vi "Input 3.vi"(8 "error in (no error)":errorcluster, 11 "Node Ptr":T2 format="%.0x") -> (0 "error out":errorcluster)   [LabVIEW 2019, in "Software Multi-Plex System Explorer.lvlib"]
uses:
  Software Multi-Plex System Explorer.lvlib
  <vilib>/NI VeriStand/Custom Device API/Custom Device Item Ref.ctl
  <vilib>/NI VeriStand/UI Controls/Tree and Alias Browser/Tree Alias Browser Display.ctl
  NationalInstruments.VeriStand.SystemStorageUI
  NationalInstruments.VeriStand.SystemStorage
  <vilib>/NI VeriStand/Custom Device API/Custom Device API.lvlib
  <vilib>/NI VeriStand/UI Controls/Tree and Alias Browser/NI_VS UI Tree Alias Browser.lvlib
panel:
  in  "Map Input":bool
  out "Input Path":string
  in  "Tree Browser":T1
  in  "Specific Header":cluster{"Section Name":string}={"Section Name"="Specify Input 3 Channel Source"}
  in  "General Header":cluster{"Section Name":string}={"Section Name"="Software Multi-Plex Channel Input 3 Settings"}
  in  "Description":string
  in  "Name":string
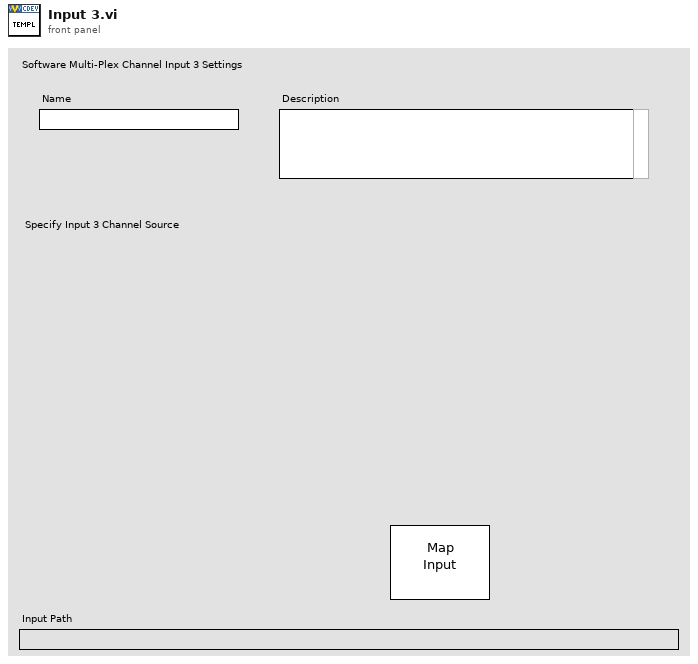
[diagram p1: front panel]
types:
  T1 = typedef "NI_VS UI Tree Alias Browser.lvlib/Tree Alias Browser Display.ctl" = refnum<k24>
  T2 = typedef "Custom Device API.lvlib/Custom Device Item Ref.ctl" = u64
  T3 = typedef "NI_VS UI Tree Alias Browser.lvlib/Callback Type.ctl" = cluster{"Net Callbacks":refnum<k27>[], "Event":T4}
  T4 = typedef "NI_VS UI Tree Alias Browser.lvlib/Net Event Data Ref.ctl" = refnum<user-event>
  T5 = typedef "NI_VS UI Tree Alias Browser.lvlib/Tree Alias Browser Ref.ctl" = refnum<k24>
  T6 = typedef "Custom Device API.lvlib/Custom Device Item Info.ctl" = cluster{"Name":string, "Is Channel":bool, "GUID":string, "Is Waveform":bool}
  T7 = typedef "Custom Device API.lvlib/Custom Device Commands.ctl" = enum16{"Default", "Item renamed", "Shutdown", "Dynamic button pressed"}
  T8 = typedef "NI_VS UI Tree Alias Browser.lvlib/Net Event.ctl" = enum16{"SelectedItem", "DblClick"}
  T9 = typedef "Custom Device API.lvlib/Custom Device Pointer.ctl" = refnum<k24>
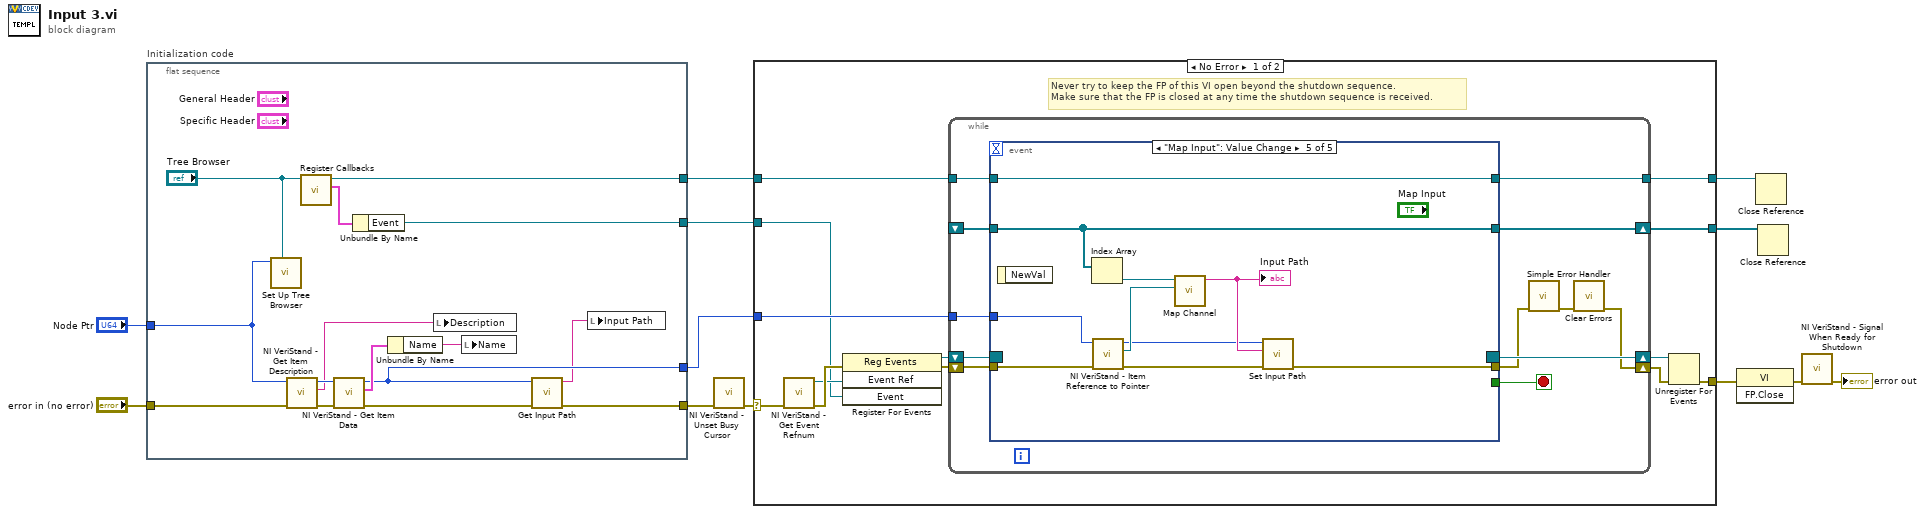
[diagram p0: block diagram]
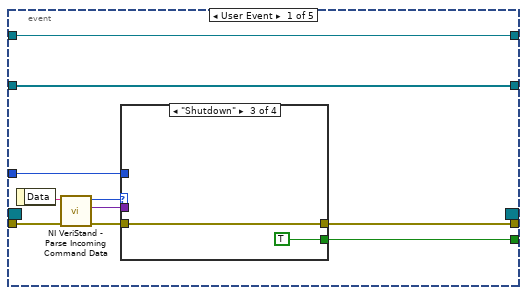
[diagram p2: hidden frame]
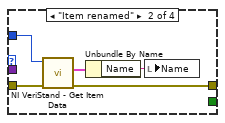
[diagram p4: hidden frame]
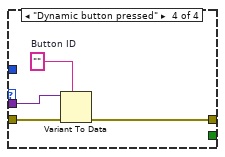
[diagram p5: hidden frame]
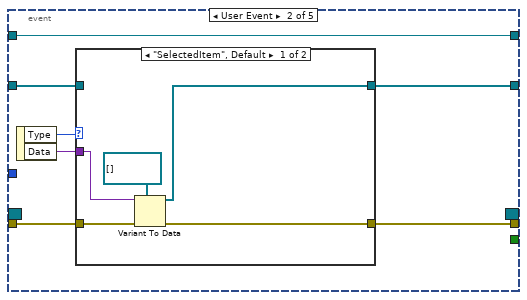
[diagram p6: hidden frame]
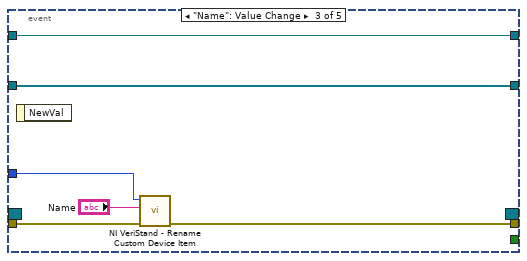
[diagram p8: hidden frame]
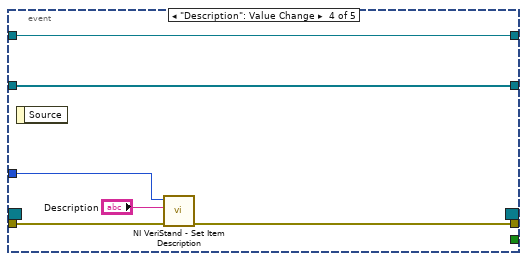
[diagram p9: hidden frame]
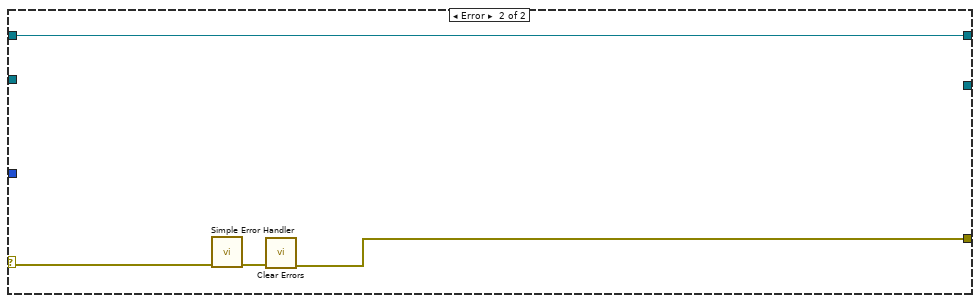
[diagram p10: hidden frame]
diagram:
  n1 = flat-sequence "Initialization code" {
    tunnel: "error in (no error)" -> [w22]
    tunnel: "Node Ptr" -> [w21]
    tunnel: [w16] -> w8
    tunnel: [w14] -> w5
    tunnel: [w19] -> w4
    tunnel: [w17] -> w2
    frame #0 {
      n2 = call "Set Up Tree Browser.vi"("Tree Ref"="Tree Browser", "Item Ref in"=w21) -> ()  [unwired: 10 in]
      n3 = call <vilib>:"NI VeriStand - Get Item Description.vi"("error in (no error)"=w22, "Item Ref in"=w21) -> ("error out"=w26:errorcluster, "Description"=w23:string, "Item Ref out"=w27:T2)  [unwired: 7 out]
      n4 = call <vilib>:"Register Callbacks.vi"("Tree Alias"="Tree Browser") -> ("Callbacks"=w18:T3, "Tree Alias dup"=w19:T5)  [unwired: 8 in, 1 out]
      n5 = call <vilib>:"NI VeriStand - Get Item Data.vi"("error in (no error)"=w26, "Item Ref in"=w27) -> ("error out"=w15:errorcluster, "Item Info"=w25:T6, "Item Ref out"=w14:T2)  [unwired: 7 out]
      n6 = Unbundle By Name(w18) -> ("Event"=w17:T4)
      n7 = Unbundle By Name(w25) -> ("Name"=w24:string)
      n8 = local write "Description"(w23) -> ()
      n9 = local write "Name"(w24) -> ()
      n10 = call "Get Input Path.vi"("error in (no error)"=w15, "Item Ref in"=w14) -> ("error out"=w16:errorcluster, "Input Path"=w13:string)  [unwired: 8 in]
      n11 = local write "Input Path"(w13) -> ()
    }
  }
  n12 = call <vilib>:"NI VeriStand - Unset Busy Cursor.vi"("error in (no error)"=w8) -> ("error out"=w7:errorcluster)  [unwired: 10 out]
  n13 = case shown="No Error" w7 {
    selector: w7 -> [w32 w114]
    tunnel: [w37 w112] -> w12
    tunnel: w5 -> [w33 _]
    tunnel: w4 -> [w31 w111]
    tunnel: [w30 w111] -> w3
    tunnel: w2 -> [w29 _]
    tunnel: [w28 _] -> w1
    frame No Error {
      # "Never try to keep the FP of this VI open beyond the shutdown sequence.\nMake sure that the FP is closed at any time the shutdown sequence is received."
      n14 = call <vilib>:"NI VeriStand - Get Event Refnum.vi"("error in (no error)"=w32) -> ("error out"=w40:errorcluster, "Event Ref"=w36:refnum<user-event>)  [unwired: 9 out]
      n15 = register-events(error in=w40, w36, w29) -> (reference out=w34:refnum<event-registration>, error out=w35:errorcluster)  [unwired: 1 in]
      n16 = while {
        tunnel: w33 -> [w48]
        shift-right: [w45] -> w38
        shift-left: w35 -> [w51]
        shift-right: [w52] -> w39
        shift-left: w34 -> [w50]
        tunnel: w31 -> [w44]
        tunnel: [w43] -> w30
        shift-right: [w42] -> w28
        shift-left: _ -> [w41]
        stop <- w49 stop-if-true
        n17 = event shown="[4] \"Map Input\": Value Change" {
          selector: w50 -> [_ _ _ _ _]
          dyn-events: [_ _ _ _ _] -> w52
          timeout: _ -> [_ _ _ _ _]
          tunnel: w51 -> [w62 w79 w94 w99 w107]
          tunnel: [w58 _ _ _ _] -> w49
          tunnel: [w57 w78 w93 w98 w104] -> w47
          tunnel: w48 -> [w56 _ w92 w100 w106]
          tunnel: w44 -> [w54 w75 w90 w96 w110]
          tunnel: [w54 w75 w90 w96 w110] -> w43
          tunnel: [w53 w77 w89 w95 w109] -> w42
          tunnel: w41 -> [w53 w76 w89 w95 w109]
          event User Event {
            n18 = event-data() -> ("Data"=w61:string)  [unwired: 1 out]
            n19 = call <vilib>:"NI VeriStand - Parse Incoming Command Data.vi"("error in (no error)"=w62, "Incoming data"=w61) -> ("error out"=w60:errorcluster, "Outgoing data"=w55:variant, "Action"=w59:T7)  [unwired: 7 out]
            n20 = case shown="\"Shutdown\"" w59 {
              tunnel: w60 -> [w63 w68 w69 w74]
              tunnel: [_ _ TRUE _] -> w58
              tunnel: [w63 w65 w69 w71] -> w57
              tunnel: w56 -> [_ w67 _ _]
              tunnel: w55 -> [_ _ _ w73]
              frame "Default", Default {
              }
              frame "Item renamed" {
                n21 = call <vilib>:"NI VeriStand - Get Item Data.vi"("error in (no error)"=w68, "Item Ref in"=w67) -> ("error out"=w65:errorcluster, "Item Info"=w66:T6)  [unwired: 8 out]
                n22 = Unbundle By Name(w66) -> ("Name"=w64:string)
                n23 = local write "Name"(w64) -> ()
              }
              frame "Shutdown" {
              }
              frame "Dynamic button pressed" {
                w72 = ""  # Button ID
                n24 = Variant To Data(error in=w74, type=w72, Variant=w73) -> (error out=w71:errorcluster)  [unwired: 1 out]
              }
            }
          }
          event User Event {
            n25 = event-data() -> ("Type"=w81:T8, "Data"=w80:variant)  [unwired: 1 out]
            n26 = case shown="\"SelectedItem\", Default" w81 {
              tunnel: w80 -> [w85 _]
              tunnel: w79 -> [w86 w87]
              tunnel: [w83 w87] -> w78
              tunnel: [w82 w88] -> w77
              tunnel: w76 -> [_ w88]
              frame "SelectedItem", Default {
                n27 = Variant To Data(error in=w86, type=refnum<k24>[] [], Variant=w85) -> (data=w82:refnum<k24>[], error out=w83:errorcluster)
              }
              frame "DblClick" {
              }
            }
          }
          event "Name": Value Change {
            n28 = event-data() -> ()  [unwired: 2 out]
            n29 = call <vilib>:"NI VeriStand - Rename Custom Device Item.vi"("error in (no error)"=w94, "New Name"="Name", "Item Ref in"=w92) -> ("error out"=w93:errorcluster)  [unwired: 1 in, 7 out]
          }
          event "Description": Value Change {
            n30 = event-data() -> ()  [unwired: 2 out]
            n31 = call <vilib>:"NI VeriStand - Set Item Description.vi"("error in (no error)"=w99, "Description"="Description", "Item Ref in"=w100) -> ("error out"=w98:errorcluster)  [unwired: 8 out]
          }
          event "Map Input": Value Change {
            n32 = event-data() -> ()  [unwired: 2 out]
            n33 = Index Array(array=w109) -> (element=w108:refnum<k24>)  [unwired: 1 in]
            n34 = call <vilib>:"NI VeriStand - Item Reference to Pointer.vi"("error in (no error)"=w107, "Item Ref in"=w106) -> ("error out"=w103:errorcluster, "Node Pointer"=w105:T9, "Item Ref out"=w101:T2)  [unwired: 6 in, 1 out]
            n35 = call "Map Channel.vi"("Destination"=w105, "Source"=w108) -> ("Source Path"=w102:string)  [unwired: 8 in, 1 out]
            "Input Path" <- w102
            n36 = call "Set Input Path.vi"("error in (no error)"=w103, "Input Path"=w102, "Item Ref in"=w101) -> ("error out"=w104:errorcluster)  [unwired: 8 in]
          }
        }
        n37 = call <vilib>:"Simple Error Handler.vi"("error in (no error)"=w47) -> ("error out"=w46:errorcluster)  [unwired: 1 in, 7 out]
        n38 = call <vilib>:"Clear Errors.vi"("error in (no error)"=w46) -> ("error out"=w45:errorcluster)  [unwired: 1 in, 5 out]
      }
      n39 = Unregister For Events(event registration refnum=w39, error in=w38) -> (error out=w37:errorcluster)
    }
    frame Error {
      n40 = call <vilib>:"Simple Error Handler.vi"("error in (no error)"=w114) -> ("error out"=w113:errorcluster)  [unwired: 1 in, 7 out]
      n41 = call <vilib>:"Clear Errors.vi"("error in (no error)"=w113) -> ("error out"=w112:errorcluster)  [unwired: 1 in, 5 out]
    }
  }
  n42 = invoke class="VI" method="FP.Close"(error in=w12) -> (error out=w11:errorcluster)  [unwired: 2 in, 2 out]
  n43 = Close Reference(reference=w3) -> ()  [unwired: 1 in, 1 out]
  n44 = Close Reference(reference=w1) -> ()  [unwired: 1 in, 1 out]
  n45 = call <vilib>:"NI VeriStand - Signal When Ready for Shutdown.vi"("error in (no error)"=w11) -> ("error out"=→"error out":errorcluster)  [unwired: 10 out]
